vi "Pockels Cal-Add header info.vi"(9 "Cal subset indexes info":string[][](array[string])=[["Cal subset indexes", ""], ["0", "11"]], 11 "Calibration data array (inc. data header row)":string[][](array[string])=[["Pockels V", "No objective", "Olympus 20X", "Nikon 25X", "Olympus 40X", "Olympus 60X"], ["0.0", "0", "", "", "", ""], ["0.1", "1.0", "", "", "", ""], ["0.2", "1.0", "", "", "", ""], ["0.3", "2.0", "", "", "", ""], ["0.4", "2.0", "", "", "", ""], ["0.5", "2.0", "", "", "", ""], ["0.6", "2.0", "", "", "", ""], ["0.7", "1.0", "", "", "", ""], ["0.8", "2.0", "", "", "", ""], ["0.9", "3.0", "", "", "", ""], ["1.0", "4.0", "", "", "", ""], ["1.1", "4.0", "", "", "", ""], ["1.2", "3.0", "", "", "", ""], ["1.3", "3.0", "", "", "", ""], ["1.4", "3.0", "", "", "", ""], ["1.5", "3.0", "", "", "", ""], ["1.6", "3.0", "", "", "", ""], ["1.7", "3.0", "", "", "", ""], ["1.8", "3.0", "", "", "", ""], ["1.9", "3.0", "", "", "", ""], ["2.0", "3.0", "", "", "", ""]]) -> (2 "Cal table (Final format)":string[][](array[string]))   [LabVIEW 2013]
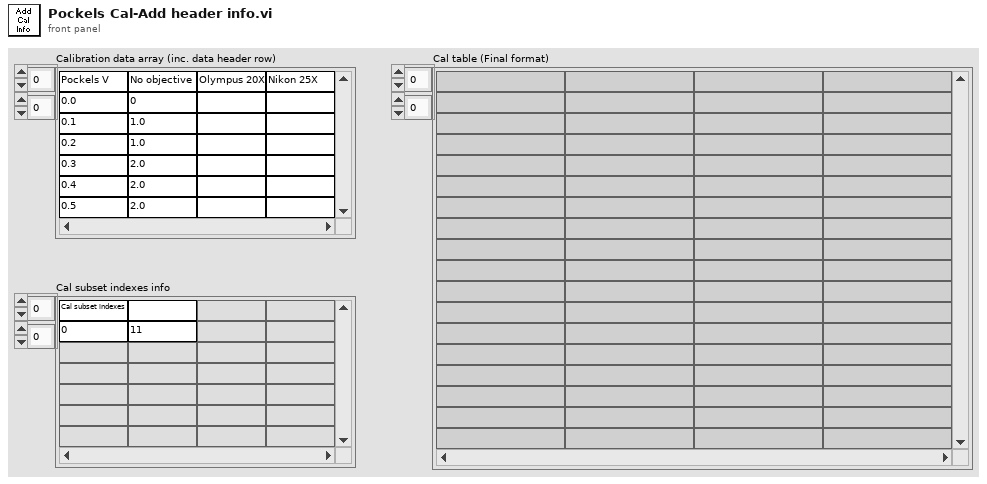
[diagram p1: front panel]
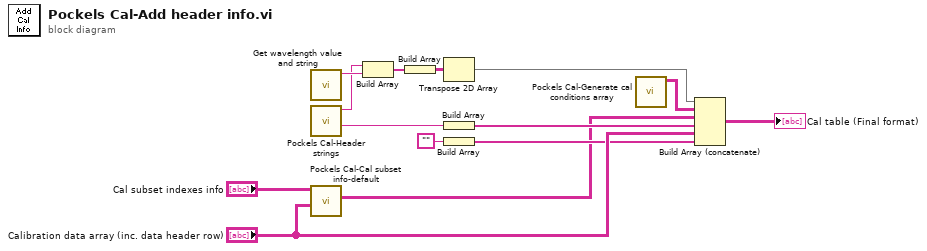
[diagram p0: block diagram]
diagram:
  n1 = call "Get wavelength value and string.vi"() -> ("Wavelength value string"=w4:string)  [unwired: 9 in, 2 out]
  n2 = call "Pockels Cal-Header strings.vi"() -> ("Cal data header string"=w11:string, "Cal wavelength string"=w3:string)  [unwired: 9 in, 1 out]
  n3 = call "Pockels Cal-Cal subset info-default.vi"("Calibration data array (inc. data header row)"="Calibration data array (inc. data header row)", "Cal subset indexes info"="Cal subset indexes info") -> ("Cal subset info array"=w5:string[][])  [unwired: 9 in]
  n4 = Build Array(w3, w4) -> (w7:string[])
  n5 = Build Array(w7) -> (w6:string[][])
  n6 = Transpose 2D Array(2D array=w6) -> (transposed array=w2:string[][])
  n7 = Build Array(w11) -> (w8:string[])
  n8 = Build Array("" ("Empty String Constant")) -> (w10:string[])
  n9 = call "Pockels Cal-Generate cal conditions array.vi"() -> ("Pockels cal conditions array"=w1:string[][])  [unwired: 11 in]
  n10 = Build Array (concatenate)(w2, w1, w5, w8, "Calibration data array (inc. data header row)", w10) -> (→"Cal table (Final format)":string[][])
